vi "SDCP SMF Tx Logger - Notifier FGV.vi"() -> ()   [LabVIEW 2020]
panel:
  in  "Commands":T1(ring)
  out "error out":errorcluster
  in  "error in (no error)":errorcluster
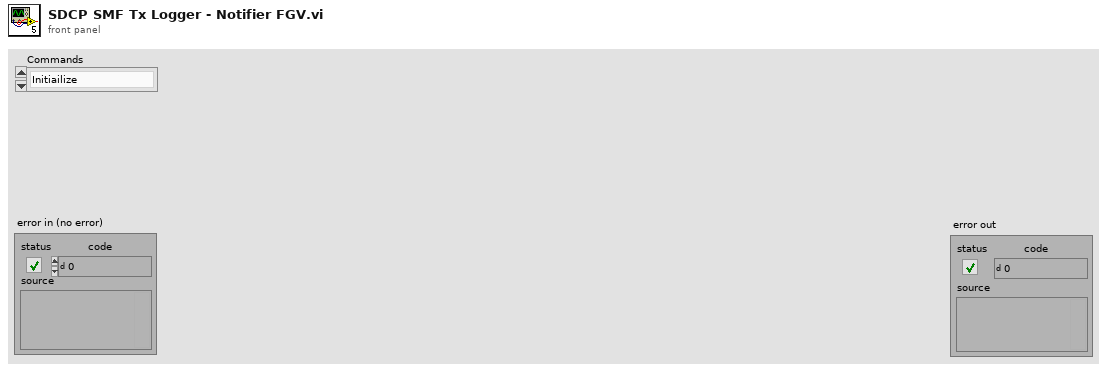
[diagram p1: front panel]
types:
  T1 = enum16{"Initiailize", "Read", "Write", "Deinitiailize"}
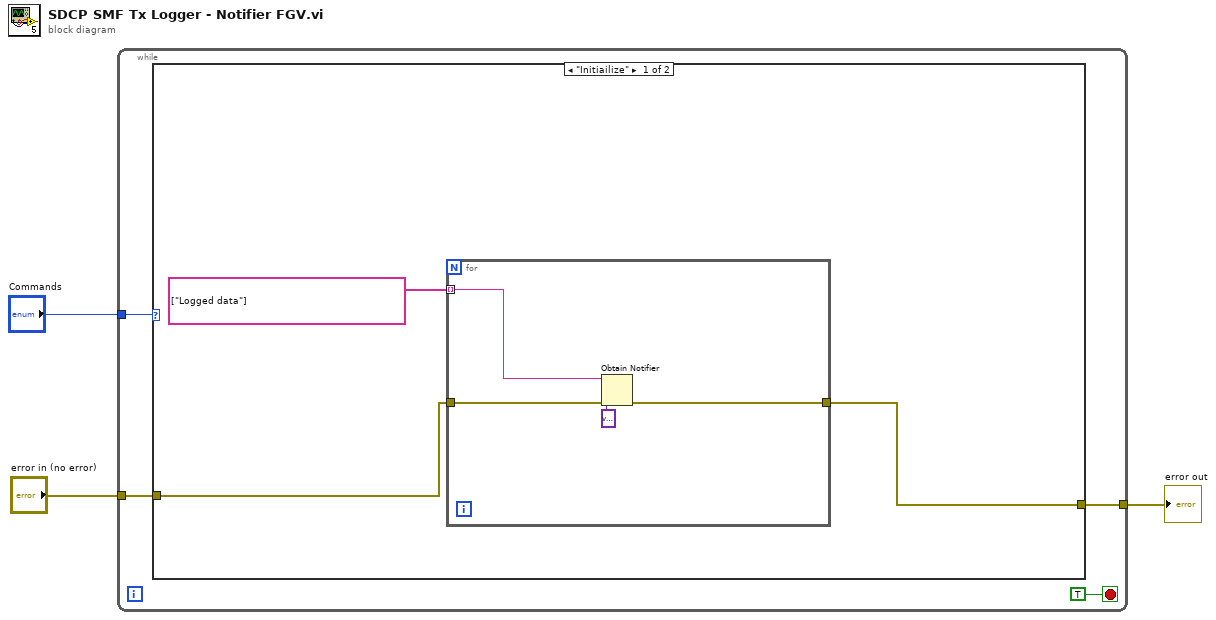
[diagram p0: block diagram]
diagram:
  n1 = while {
    tunnel: "error in (no error)" -> [w5]
    tunnel: "Commands" -> [w6]
    tunnel: [w4] -> w1
    stop <- TRUE stop-if-true
    n2 = case shown="\"Initiailize\"" w6 {
      tunnel: w5 -> [w10 _]
      tunnel: [w9 _] -> w4
      frame "Initiailize" {
        n3 = for {
          tunnel: w10 -> [w14]
          tunnel: [w13] -> w9
          tunnel: string[] ["Logged data"] -> [w12] mode=indexing
          n4 = Obtain Notifier(name (unnamed)=w12, notification data type=variant ("element data type"), error in (no error)=w14) -> (error out=w13:errorcluster)  [unwired: 1 in, 2 out]
        }
      }
      frame "Read" {
      }
    }
  }
  "error out" <- w1
